vi "ConfFileParser.vi"(0 "TEXT":string, 1 "search string":string) -> (2 "Cluster Array":T1(array[cluster]), 3 "Names":string[](array[string]), 4 "Codes":string[](array[string]))   [LabVIEW 2009]
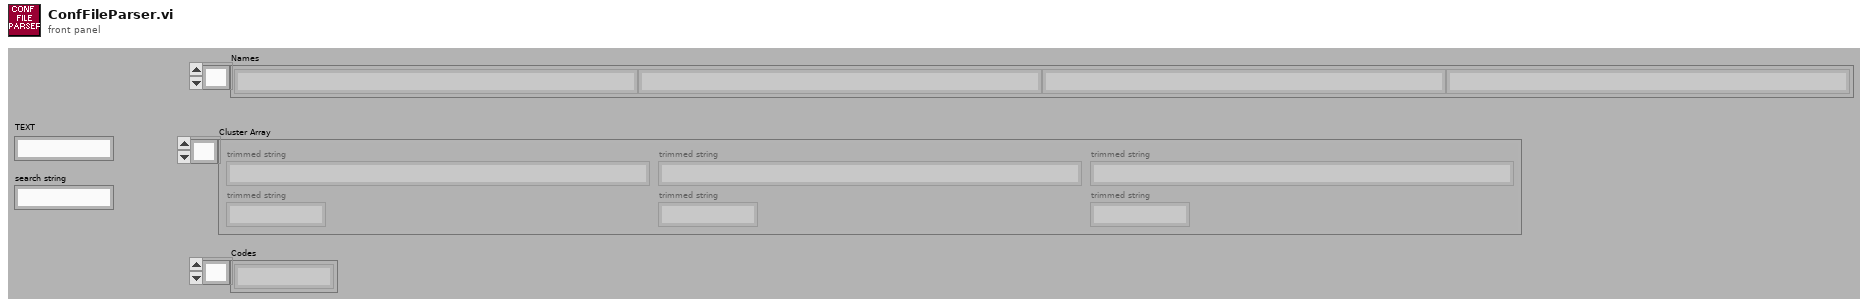
[diagram p1: front panel]
types:
  T1 = cluster{"trimmed string":string, "trimmed string":string}[]
  T2 = cluster{"trimmed string":string, "trimmed string":string}
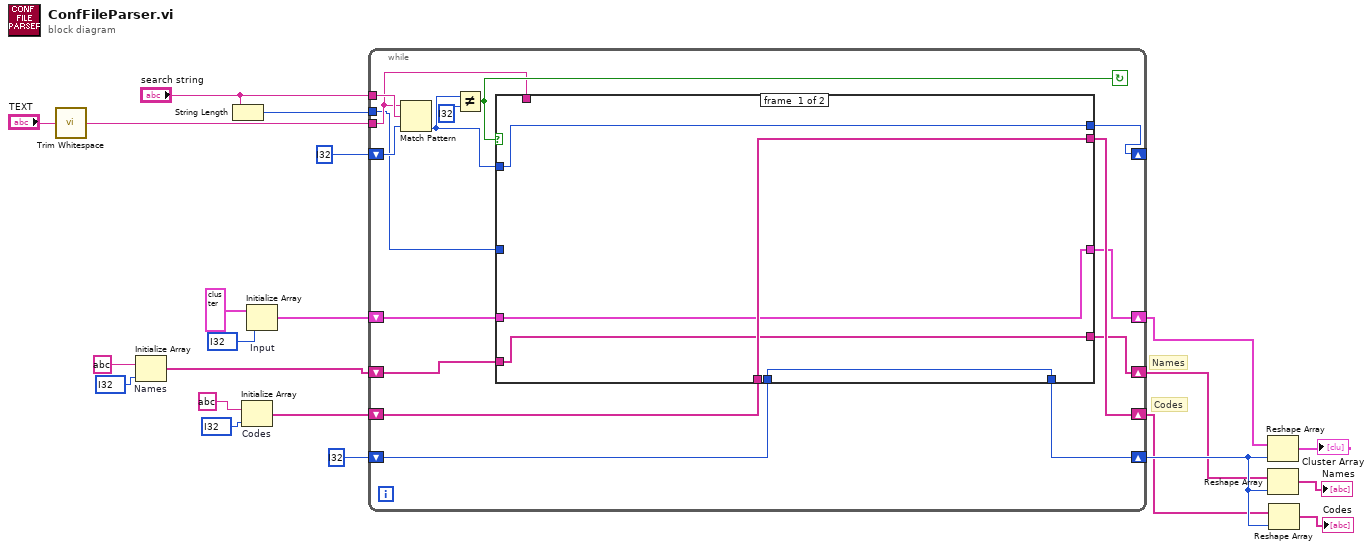
[diagram p0: block diagram]
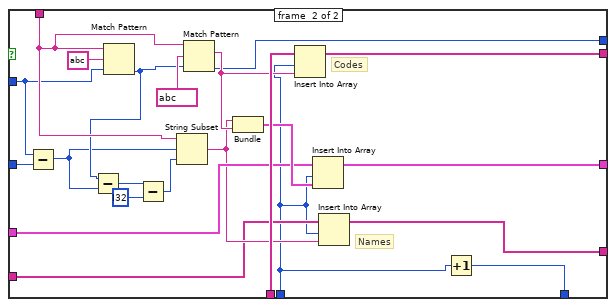
[diagram p2: hidden frame]
diagram:
  # "Names"
  # "Codes"
  n1 = call <vilib>:"Trim Whitespace.vi"("string"="TEXT") -> ("trimmed string"=w13:string)  [unwired: 1 in]
  n2 = Initialize Array "Names"(string ? ("trimmed string"), i32 ? ("dimension size")) -> (w14:string[])
  n3 = String Length(string="search string") -> (length=w9:i32)
  n4 = Initialize Array "Codes"(string ? ("trimmed string"), i32 ? ("dimension size")) -> (w11:string[])
  n5 = Initialize Array "Input"(T2 ? ("output cluster"), i32 ? ("dimension size")) -> (w15:T1)
  n6 = while {
    tunnel: "search string" -> [w36]
    tunnel: w13 -> [w34]
    shift-right: [w29] -> _
    shift-left: i32 ? ("offset (0)") -> [w31]
    shift-right: [w26] -> w6
    shift-left: w15 -> [w27]
    shift-right: [w23] -> w4
    shift-left: w14 -> [w25]
    shift-right: [w32] -> w3
    shift-left: w11 -> [w33]
    tunnel: w9 -> [w30]
    shift-right: [w24] -> w7
    shift-left: i32 ? ("dimension size") -> [w28]
    stop <- w37 continue-if-true
    n7 = Match Pattern(string=w34, regular expression=w36, offset (0)=w31) -> (offset past match=w35:i32)  [unwired: 3 out]
    n8 = Not Equal?(x=w35, y=i32 ?) -> (x != y?=w37:bool)
    n9 = case shown="True" w37 {
      tunnel: w34 -> [_ w60]
      tunnel: w35 -> [w42 w59]
      tunnel: w33 -> [w43 w63]
      tunnel: [w43 w62] -> w32
      tunnel: w30 -> [_ w48]
      tunnel: [w42 w57] -> w29
      tunnel: w28 -> [w41 w51]
      tunnel: w27 -> [w40 w55]
      tunnel: [w40 w54] -> w26
      tunnel: w25 -> [w39 w52]
      tunnel: [w41 w50] -> w24
      tunnel: [w39 w49] -> w23
      frame #0 {
      }
      frame #1 {
        # "Names"
        # "Codes"
        n10 = Subtract(x=w59, y=w48) -> (x-y=w47:i32)
        n11 = Match Pattern(string=w60, regular expression=string ? ("search string"), offset (0)=w59) -> (offset past match=w58:i32)  [unwired: 3 out]
        n12 = Subtract(x=w58, y=w47) -> (x-y=w45:i32)
        n13 = Subtract(x=w45, y=i32 ?) -> (x-y=w44:i32)
        n14 = String Subset(string=w60, offset (0)=w47, length (rest)=w44) -> (substring=w53:string)
        n15 = Match Pattern(string=w60, regular expression=string ?, offset (0)=w58) -> (match substring=w61:string, offset past match=w57:i32)  [unwired: 2 out]
        n16 = Bundle("trimmed string"=w53, "trimmed string"=w61) -> (w56:T2)  [unwired: 1 in]
        n17 = Insert Into Array(array=w63, index=w51, new element=w61) -> (w62:string[])
        n18 = Insert Into Array(array=w55, index=w51, new element=w56) -> (w54:T1)
        n19 = Insert Into Array(array=w52, index=w51, new element=w53) -> (w49:string[])
        n20 = Increment(x=w51) -> (x+1=w50:i32)
      }
    }
  }
  n21 = Reshape Array(w6, w7) -> (→"Cluster Array":T1)
  n22 = Reshape Array(w4, w7) -> (→"Names":string[])
  n23 = Reshape Array(w3, w7) -> (→"Codes":string[])
